vi "CreateControlPanel_ExtSensors.vi"(6 "MODE (A/DIO13 (Pin 26))":bool, 7 "Speed (P2) (A/AI0 (Pin 3))":dbl, 8 "MOVE RIGHT (E3) (A/DIO3 (Pin 17))":bool, 9 "MOVE LEFT (E3) (A/DIO2 (Pin 15))":bool, 10 "TETHER IN (P2) (A/DIO1 (Pin 13))":bool, 11 "TETHER OUT (P2) (A/DIO0 (Pin 11))":bool) -> (3 "Control Panel (EXT. CONTROLS)":T1={"Speed"=1, "Tether Control"=enum."Radio Selection 2", "Pulley Control"=enum."Radio Selection 2", "Mode"=enum."Radio Selection 1"} {"Speed" scale=0.0..2.0})   [LabVIEW 2018]
uses:
  Custom Controls/ControlPanel.ctl
panel:
  # "NORMAL"
  # "SLOW"
  # "FAST"
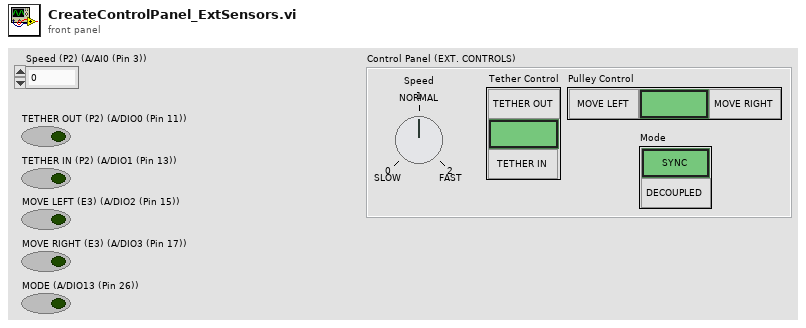
[diagram p1: front panel]
types:
  T1 = typedef "ControlPanel.ctl" = cluster{"Speed":u8, "Tether Control":enum32{"Radio Selection 1", "Radio Selection 2", "Radio Selection 3"}, "Pulley Control":enum32{"Radio Selection 1", "Radio Selection 2", "Radio Selection 3"}, "Mode":enum32{"Radio Selection 1", "Radio Selection 2"}}
  T2 = enum32{"Radio Selection 1", "Radio Selection 2", "Radio Selection 3"}
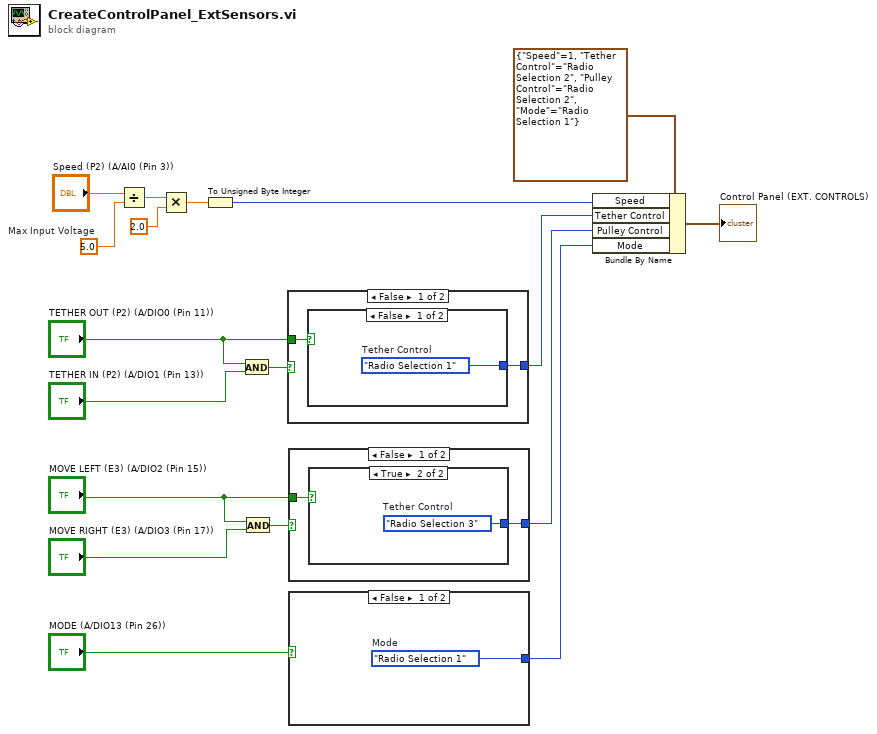
[diagram p0: block diagram]
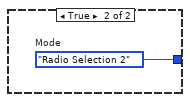
[diagram p2: hidden frame]
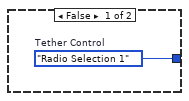
[diagram p3: hidden frame]
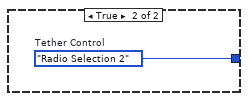
[diagram p4: hidden frame]
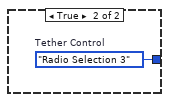
[diagram p5: hidden frame]
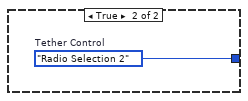
[diagram p6: hidden frame]
diagram:
  w17 = 5.0  # Max Input Voltage
  n1 = Divide(x="Speed (P2) (A/AI0 (Pin 3))", y=w17) -> (x/y=w16:dbl)
  n2 = Multiply(x=w16, y=2.0) -> (x*y=w14:dbl)
  n3 = To Unsigned Byte Integer(number=w14) -> (unsigned 8bit integer=w12:u8)
  n4 = And(x="TETHER OUT (P2) (A/DIO0 (Pin 11))", y="TETHER IN (P2) (A/DIO1 (Pin 13))") -> (x .and. y?=w9:bool)
  n5 = And(x="MOVE LEFT (E3) (A/DIO2 (Pin 15))", y="MOVE RIGHT (E3) (A/DIO3 (Pin 17))") -> (x .and. y?=w6:bool)
  n6 = case shown="False" w9 {
    tunnel: [w19 w23] -> w7
    tunnel: "TETHER OUT (P2) (A/DIO0 (Pin 11))" -> [w20 _]
    frame False {
      n7 = case shown="False" w20 {
        tunnel: [w21 w22] -> w19
        frame False {
          w21 = T2."Radio Selection 1"  # Tether Control
        }
        frame True {
          w22 = T2."Radio Selection 3"  # Tether Control
        }
      }
    }
    frame True {
      w23 = T2."Radio Selection 2"  # Tether Control
    }
  }
  n8 = case shown="False" w6 {
    tunnel: [w24 w28] -> w3
    tunnel: "MOVE LEFT (E3) (A/DIO2 (Pin 15))" -> [w25 _]
    frame False {
      n9 = case shown="True" w25 {
        tunnel: [w26 w27] -> w24
        frame False {
          w26 = T2."Radio Selection 1"  # Tether Control
        }
        frame True {
          w27 = T2."Radio Selection 3"  # Tether Control
        }
      }
    }
    frame True {
      w28 = T2."Radio Selection 2"  # Tether Control
    }
  }
  n10 = case shown="False" "MODE (A/DIO13 (Pin 26))" {
    tunnel: [w29 w30] -> w1
    frame False {
      w29 = enum32{"Radio Selection 1", "Radio Selection 2"}."Radio Selection 1"  # Mode
    }
    frame True {
      w30 = enum32{"Radio Selection 1", "Radio Selection 2"}."Radio Selection 2"  # Mode
    }
  }
  n11 = Bundle By Name(cluster=T1 {"Speed"=1, "Tether Control"=enum."Radio Selection 2", "Pulley Control"=enum."Radio Selection 2", "Mode"=enum."Radio Selection 1"} ("Control Panel (EXT. CONTROLS)"), "Speed"=w12, "Tether Control"=w7, "Pulley Control"=w3, "Mode"=w1) -> (→"Control Panel (EXT. CONTROLS)":T1)
